vi "JSONable Tests.vi"() -> ()   [LabVIEW 2015]
uses:
  Classes/error/error.lvclass
  Classes/id/id.lvclass
  Classes/Request/Request.lvclass
  Classes/Response/Response.lvclass
  Classes/params/params.lvclass
  Classes/New folder/result.lvclass
  <vilib>/National Instruments/JSON Support for LabVIEW/JSON Data Classes/JSON String/New JSON String.vi
  <vilib>/National Instruments/JSON Support for LabVIEW/JSON Data Classes/JSON Numeric/New JSON Numeric.vi
  <vilib>/National Instruments/JSON Support for LabVIEW/JSON Data Classes/JSON Array/New JSON Array (Numeric).vi
  <vilib>/National Instruments/JSON Support for LabVIEW/JSON Data Classes/JSON Object/New JSON Object (Empty).vi
  <vilib>/National Instruments/JSON Support for LabVIEW/JSON Data Classes/JSON Object/Insert Key Value Pair (Single Boolean).vi
  <vilib>/National Instruments/JSON Support for LabVIEW/JSON Data Classes/JSON Object/Insert Key Value Pair (Single Numeric).vi
  <vilib>/National Instruments/JSON Support for LabVIEW/JSON Data Classes/JSON Object/Insert Key Value Pair (Single String).vi
  <vilib>/National Instruments/JSON Support for LabVIEW/JSON Data Classes/JSON Object/Insert Key Value Pair (Single).vi
  <vilib>/National Instruments/JSON Support for LabVIEW/JSON Data Classes/JSON Datatype/New JSON Null.vi
  Classes/JSONable/JSONable.lvclass
  <vilib>/National Instruments/JSON Support for LabVIEW/JSON Data Classes/JSON Helper/JSON Helper.lvclass
  <vilib>/National Instruments/JSON Support for LabVIEW/JSON Data Classes/JSON String/JSON String.lvclass
  <vilib>/National Instruments/JSON Support for LabVIEW/JSON Data Classes/JSON Array/JSON Array.lvclass
  <vilib>/National Instruments/JSON Support for LabVIEW/JSON Data Classes/JSON Numeric/JSON Numeric.lvclass
  <vilib>/National Instruments/JSON Support for LabVIEW/JSON Data Classes/JSON Object/JSON Object.lvclass
  <vilib>/National Instruments/JSON Support for LabVIEW/JSON Data Classes/JSON Datatype/JSON Null.lvclass
panel:
  out "result(String)":bool
  out "params(String)":bool
  out "result(named and nested)":bool
  out "result(DBL Array)":bool
  out "no result":bool
  out "response (error)":bool
  out "response (result)":bool
  out "notification":bool
  out "request (named params)":bool
  out "request (array params)":bool
  out "params(named and nested)":bool
  out "params(DBL Array)":bool
  out "no params":bool
  out "id(none)":bool
  out "id(NULL)":bool
  out "id(String)":bool
  out "id(Double)":bool
  out "error":bool
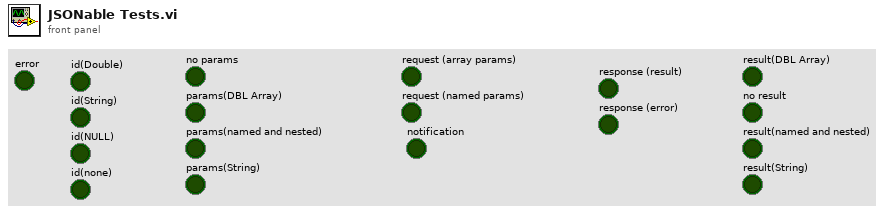
[diagram p1: front panel]
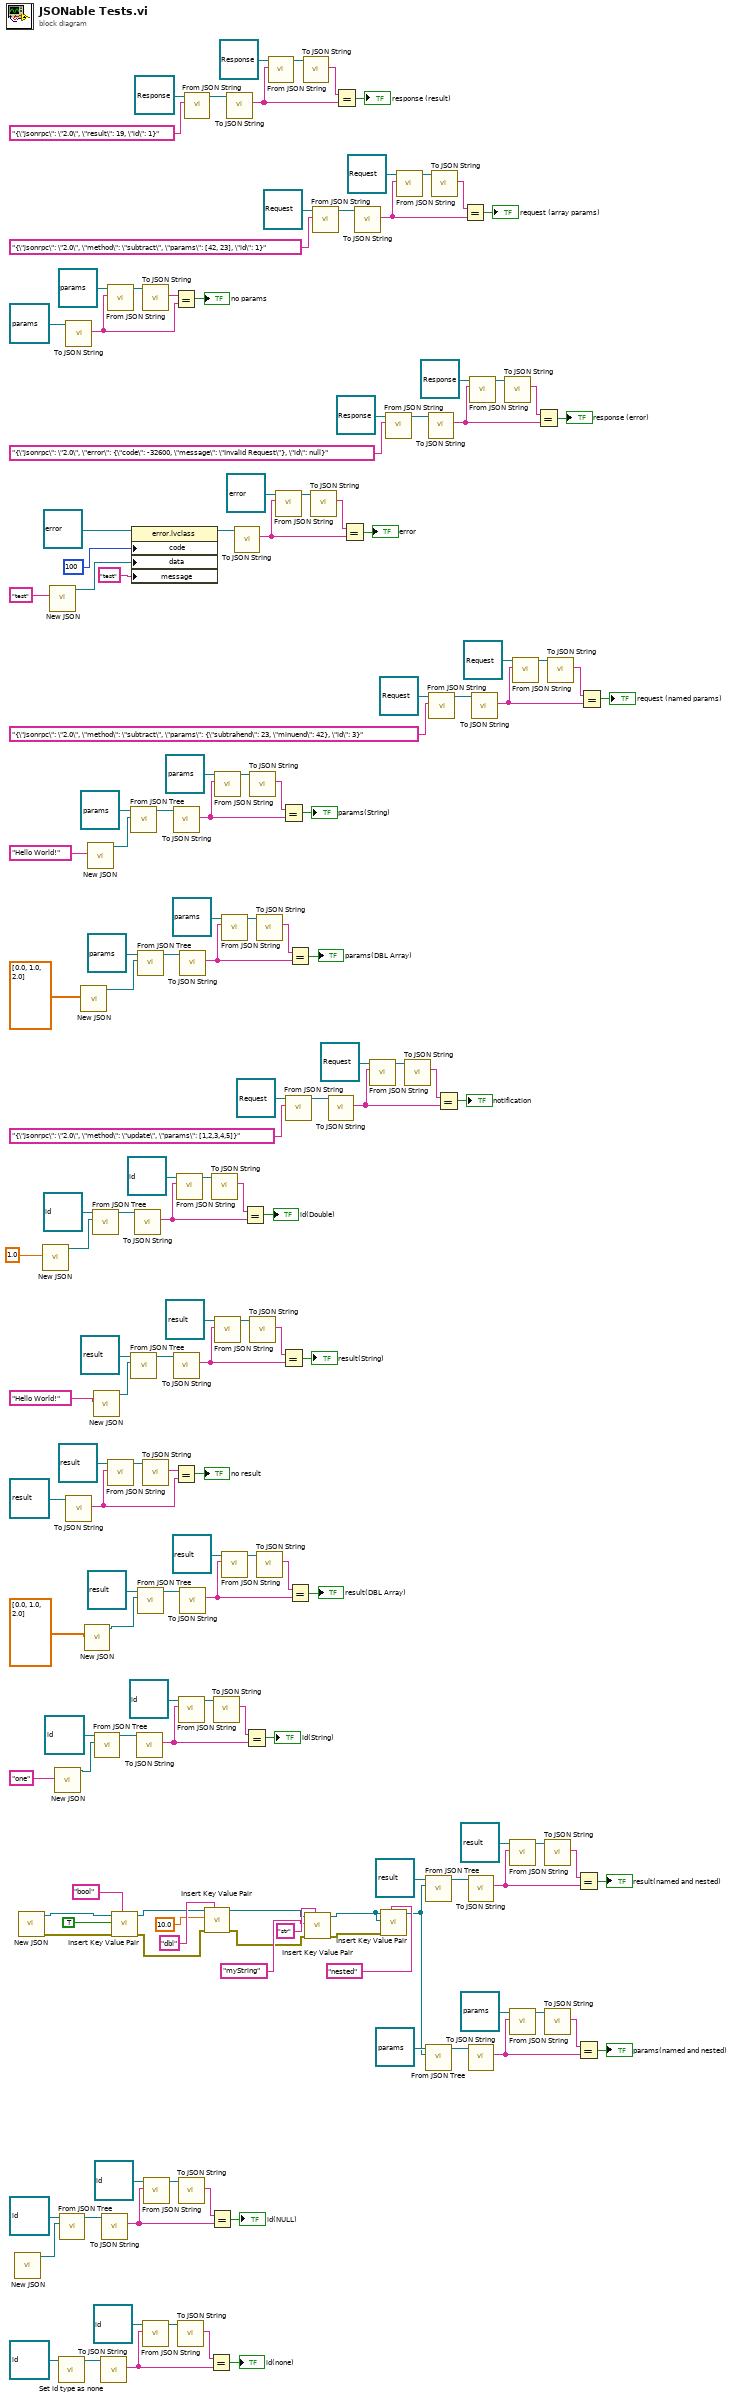
[diagram p0: block diagram]
diagram:
  n1 = call-poly <vilib>:"New JSON.vi"() -> ("JSON Null out"=w1:refnum<class "JSON Null.lvclass">)  [unwired: 10 in, 1 out]
  n2 = call-poly <vilib>:"New JSON.vi"() -> ("error out"=w14:errorcluster, "JSON Object out"=w15:refnum<class "JSON Object.lvclass">)  [unwired: 10 in]
  n3 = call-poly <vilib>:"New JSON.vi"("value"=1.0 ("Numeric")) -> ("JSON String out"=w132:refnum<class "JSON Numeric.lvclass">)  [unwired: 9 in, 1 out]
  n4 = call-poly <vilib>:"New JSON.vi"("value"="test" ("String")) -> ("JSON String out"=w145:refnum<class "JSON String.lvclass">)  [unwired: 9 in, 1 out]
  n5 = call-poly <vilib>:"New JSON.vi"("value"="one" ("String")) -> ("JSON String out"=w18:refnum<class "JSON String.lvclass">)  [unwired: 9 in, 1 out]
  n6 = call-dynamic "Set id type as none.vi"("id in"=refnum<class "id.lvclass"> refnum ("id.lvclass")) -> ("id out"=w156:refnum<class "id.lvclass">)  [unwired: 9 in, 1 out]
  n7 = call-dynamic "From JSON Tree.vi"("JSON in"=w1, "id in"=refnum<class "id.lvclass"> refnum ("id.lvclass")) -> ("id out"=w118:refnum<class "id.lvclass">)  [unwired: 8 in, 1 out]
  n8 = call "To JSON String.vi"("JSONable in"=refnum<class "params.lvclass"> refnum ("params.lvclass")) -> ("JSON String"=w154:string)  [unwired: 8 in, 2 out]
  n9 = call "To JSON String.vi"("JSONable in"=refnum<class "result.lvclass"> refnum ("result.lvclass")) -> ("JSON String"=w58:string)  [unwired: 8 in, 2 out]
  n10 = call-poly <vilib>:"New JSON.vi"("Numeric Array"=dbl[] [0.0, 1.0, 2.0] ("1D Numeric")) -> ("JSON Array out"=w110:refnum<class "JSON Array.lvclass">)  [unwired: 9 in, 1 out]
  n11 = call-poly <vilib>:"New JSON.vi"("Numeric Array"=dbl[] [0.0, 1.0, 2.0] ("1D Numeric")) -> ("JSON Array out"=w20:refnum<class "JSON Array.lvclass">)  [unwired: 9 in, 1 out]
  n12 = call-poly <vilib>:"New JSON.vi"("value"="Hello World!" ("String")) -> ("JSON String out"=w41:refnum<class "JSON String.lvclass">)  [unwired: 9 in, 1 out]
  n13 = call-dynamic "From JSON Tree.vi"("JSON in"=w132, "id in"=refnum<class "id.lvclass"> refnum ("id.lvclass")) -> ("id out"=w131:refnum<class "id.lvclass">)  [unwired: 8 in, 1 out]
  n14 = call-poly <vilib>:"New JSON.vi"("value"="Hello World!" ("String")) -> ("JSON String out"=w22:refnum<class "JSON String.lvclass">)  [unwired: 9 in, 1 out]
  n15 = call-dynamic "From JSON Tree.vi"("JSON in"=w18, "id in"=refnum<class "id.lvclass"> refnum ("id.lvclass")) -> ("id out"=w130:refnum<class "id.lvclass">)  [unwired: 8 in, 1 out]
  n16 = call "To JSON String.vi"("JSONable in"=w156) -> ("JSON String"=w159:string)  [unwired: 8 in, 2 out]
  n17 = call "To JSON String.vi"("JSONable in"=w118) -> ("JSON String"=w122:string)  [unwired: 8 in, 2 out]
  n18 = call "From JSON String.vi"("JSON String"=w154, "JSONable in"=refnum<class "params.lvclass"> refnum ("params.lvclass")) -> ("JSONable out"=w152:refnum<class "params.lvclass">)  [unwired: 8 in, 1 out]
  n19 = call "From JSON String.vi"("JSON String"=w58, "JSONable in"=refnum<class "result.lvclass"> refnum ("result.lvclass")) -> ("JSONable out"=w60:refnum<class "result.lvclass">)  [unwired: 8 in, 1 out]
  n20 = call-poly <vilib>:"Insert Key Value Pair.vi"("key"="bool" ("Name"), "error in (no error)"=w14, "value"=TRUE ("Boolean"), "JSON Object in"=w15) -> ("error out"=w10:errorcluster, "JSON Object out"=w11:refnum<class "JSON Object.lvclass">)  [unwired: 5 in, 1 out]
  n21 = call-dynamic "From JSON Tree.vi"("JSON in"=w41, "params in"=refnum<class "params.lvclass"> refnum ("params.lvclass")) -> ("params out"=w42:refnum<class "params.lvclass">)  [unwired: 8 in, 1 out]
  n22 = call-dynamic "From JSON Tree.vi"("JSON in"=w22, "result in"=refnum<class "result.lvclass"> refnum ("result.lvclass")) -> ("result out"=w27:refnum<class "result.lvclass">)  [unwired: 8 in, 1 out]
  n23 = property class="error.lvclass"(reference=refnum<class "error.lvclass"> refnum ("error.lvclass"), "code"=100, "data"=w145, "message"="test") -> (reference out=w148:refnum<class "error.lvclass">)  [unwired: 1 in, 1 out]
  n24 = call "To JSON String.vi"("JSONable in"=w131) -> ("JSON String"=w137:string)  [unwired: 8 in, 2 out]
  n25 = call "To JSON String.vi"("JSONable in"=w130) -> ("JSON String"=w125:string)  [unwired: 8 in, 2 out]
  n26 = call-dynamic "From JSON Tree.vi"("JSON in"=w110, "params in"=refnum<class "params.lvclass"> refnum ("params.lvclass")) -> ("params out"=w109:refnum<class "params.lvclass">)  [unwired: 8 in, 1 out]
  n27 = call-dynamic "From JSON Tree.vi"("JSON in"=w20, "result in"=refnum<class "result.lvclass"> refnum ("result.lvclass")) -> ("result out"=w56:refnum<class "result.lvclass">)  [unwired: 8 in, 1 out]
  n28 = call "To JSON String.vi"("JSONable in"=w152) -> ("JSON String"=w153:string)  [unwired: 8 in, 2 out]
  n29 = call "To JSON String.vi"("JSONable in"=w60) -> ("JSON String"=w59:string)  [unwired: 8 in, 2 out]
  n30 = call "From JSON String.vi"("JSON String"=w159, "JSONable in"=refnum<class "id.lvclass"> refnum ("id.lvclass")) -> ("JSONable out"=w161:refnum<class "id.lvclass">)  [unwired: 8 in, 1 out]
  n31 = call "From JSON String.vi"("JSON String"=w122, "JSONable in"=refnum<class "id.lvclass"> refnum ("id.lvclass")) -> ("JSONable out"=w120:refnum<class "id.lvclass">)  [unwired: 8 in, 1 out]
  n32 = Equal?(x=w153, y=w154) -> (x = y?=→"no params":bool)
  n33 = call "To JSON String.vi"("JSONable in"=w42) -> ("JSON String"=w38:string)  [unwired: 8 in, 2 out]
  n34 = call "To JSON String.vi"("JSONable in"=w27) -> ("JSON String"=w30:string)  [unwired: 8 in, 2 out]
  n35 = Equal?(x=w59, y=w58) -> (x = y?=→"no result":bool)
  n36 = call "From JSON String.vi"("JSON String"=w137, "JSONable in"=refnum<class "id.lvclass"> refnum ("id.lvclass")) -> ("JSONable out"=w135:refnum<class "id.lvclass">)  [unwired: 8 in, 1 out]
  n37 = call "To JSON String.vi"("JSONable in"=w161) -> ("JSON String"=w160:string)  [unwired: 8 in, 2 out]
  n38 = call "From JSON String.vi"("JSON String"=w125, "JSONable in"=refnum<class "id.lvclass"> refnum ("id.lvclass")) -> ("JSONable out"=w127:refnum<class "id.lvclass">)  [unwired: 8 in, 1 out]
  n39 = call "To JSON String.vi"("JSONable in"=w120) -> ("JSON String"=w121:string)  [unwired: 8 in, 2 out]
  n40 = call "To JSON String.vi"("JSONable in"=w109) -> ("JSON String"=w113:string)  [unwired: 8 in, 2 out]
  n41 = call "To JSON String.vi"("JSONable in"=w56) -> ("JSON String"=w53:string)  [unwired: 8 in, 2 out]
  n42 = call "From JSON String.vi"("JSON String"="{\"jsonrpc\": \"2.0\", \"result\": 19, \"id\": 1}", "JSONable in"=refnum<class "Response.lvclass"> refnum ("Response.lvclass")) -> ("JSONable out"=w77:refnum<class "Response.lvclass">)  [unwired: 8 in, 1 out]
  n43 = call-poly <vilib>:"Insert Key Value Pair.vi"("key"="dbl" ("Name"), "error in (no error)"=w10, "value"=10.0 ("Numeric"), "JSON Object in"=w11) -> ("error out"=w7:errorcluster, "JSON Object out"=w5:refnum<class "JSON Object.lvclass">)  [unwired: 5 in, 1 out]
  n44 = Equal?(x=w160, y=w159) -> (x = y?=→"id(none)":bool)
  n45 = Equal?(x=w121, y=w122) -> (x = y?=→"id(NULL)":bool)
  n46 = call "To JSON String.vi"("JSONable in"=w135) -> ("JSON String"=w136:string)  [unwired: 8 in, 2 out]
  n47 = call "To JSON String.vi"("JSONable in"=w127) -> ("JSON String"=w126:string)  [unwired: 8 in, 2 out]
  n48 = call "From JSON String.vi"("JSON String"=w38, "JSONable in"=refnum<class "params.lvclass"> refnum ("params.lvclass")) -> ("JSONable out"=w36:refnum<class "params.lvclass">)  [unwired: 8 in, 1 out]
  n49 = call "From JSON String.vi"("JSON String"=w30, "JSONable in"=refnum<class "result.lvclass"> refnum ("result.lvclass")) -> ("JSONable out"=w32:refnum<class "result.lvclass">)  [unwired: 8 in, 1 out]
  n50 = call "From JSON String.vi"("JSON String"=w113, "JSONable in"=refnum<class "params.lvclass"> refnum ("params.lvclass")) -> ("JSONable out"=w115:refnum<class "params.lvclass">)  [unwired: 8 in, 1 out]
  n51 = call "From JSON String.vi"("JSON String"=w53, "JSONable in"=refnum<class "result.lvclass"> refnum ("result.lvclass")) -> ("JSONable out"=w51:refnum<class "result.lvclass">)  [unwired: 8 in, 1 out]
  n52 = call "To JSON String.vi"("JSONable in"=w77) -> ("JSON String"=w72:string)  [unwired: 8 in, 2 out]
  n53 = call "To JSON String.vi"("JSONable in"=w148) -> ("JSON String"=w140:string)  [unwired: 8 in, 2 out]
  n54 = Equal?(x=w136, y=w137) -> (x = y?=→"id(Double)":bool)
  n55 = Equal?(x=w126, y=w125) -> (x = y?=→"id(String)":bool)
  n56 = call "To JSON String.vi"("JSONable in"=w36) -> ("JSON String"=w37:string)  [unwired: 8 in, 2 out]
  n57 = call "To JSON String.vi"("JSONable in"=w32) -> ("JSON String"=w31:string)  [unwired: 8 in, 2 out]
  n58 = call "To JSON String.vi"("JSONable in"=w115) -> ("JSON String"=w114:string)  [unwired: 8 in, 2 out]
  n59 = call "To JSON String.vi"("JSONable in"=w51) -> ("JSON String"=w52:string)  [unwired: 8 in, 2 out]
  n60 = call "From JSON String.vi"("JSON String"=w72, "JSONable in"=refnum<class "Response.lvclass"> refnum ("Response.lvclass")) -> ("JSONable out"=w74:refnum<class "Response.lvclass">)  [unwired: 8 in, 1 out]
  n61 = call "From JSON String.vi"("JSON String"=w140, "JSONable in"=refnum<class "error.lvclass"> refnum ("error.lvclass")) -> ("JSONable out"=w142:refnum<class "error.lvclass">)  [unwired: 8 in, 1 out]
  n62 = Equal?(x=w37, y=w38) -> (x = y?=→"params(String)":bool)
  n63 = Equal?(x=w31, y=w30) -> (x = y?=→"result(String)":bool)
  n64 = call "From JSON String.vi"("JSON String"="{\"jsonrpc\": \"2.0\", \"method\": \"update\", \"params\": [1,2,3,4,5]}", "JSONable in"=refnum<class "Request.lvclass"> refnum ("Request.lvclass")) -> ("JSONable out"=w80:refnum<class "Request.lvclass">)  [unwired: 8 in, 1 out]
  n65 = Equal?(x=w114, y=w113) -> (x = y?=→"params(DBL Array)":bool)
  n66 = Equal?(x=w52, y=w53) -> (x = y?=→"result(DBL Array)":bool)
  n67 = call "To JSON String.vi"("JSONable in"=w74) -> ("JSON String"=w73:string)  [unwired: 8 in, 2 out]
  n68 = call-poly <vilib>:"Insert Key Value Pair.vi"("key"="str" ("Name"), "error in (no error)"=w7, "value"="myString" ("String"), "JSON Object in"=w5) -> ("error out"=w6:errorcluster, "JSON Object out"=w4:refnum<class "JSON Object.lvclass">)  [unwired: 5 in, 1 out]
  n69 = call "To JSON String.vi"("JSONable in"=w142) -> ("JSON String"=w141:string)  [unwired: 8 in, 2 out]
  n70 = call "From JSON String.vi"("JSON String"="{\"jsonrpc\": \"2.0\", \"method\": \"subtract\", \"params\": [42, 23], \"id\": 1}", "JSONable in"=refnum<class "Request.lvclass"> refnum ("Request.lvclass")) -> ("JSONable out"=w95:refnum<class "Request.lvclass">)  [unwired: 8 in, 1 out]
  n71 = call "To JSON String.vi"("JSONable in"=w80) -> ("JSON String"=w85:string)  [unwired: 8 in, 2 out]
  n72 = Equal?(x=w73, y=w72) -> (x = y?=→"response (result)":bool)
  n73 = Equal?(x=w141, y=w140) -> (x = y?=→"error":bool)
  n74 = call "To JSON String.vi"("JSONable in"=w95) -> ("JSON String"=w100:string)  [unwired: 8 in, 2 out]
  n75 = call "From JSON String.vi"("JSON String"=w85, "JSONable in"=refnum<class "Request.lvclass"> refnum ("Request.lvclass")) -> ("JSONable out"=w83:refnum<class "Request.lvclass">)  [unwired: 8 in, 1 out]
  n76 = call-poly <vilib>:"Insert Key Value Pair.vi"("key"="nested" ("Name"), "error in (no error)"=w6, "value"=w4, "JSON Object in"=w4) -> ("JSON Object out"=w2:refnum<class "JSON Object.lvclass">)  [unwired: 5 in, 2 out]
  n77 = call "From JSON String.vi"("JSON String"="{\"jsonrpc\": \"2.0\", \"error\": {\"code\": -32600, \"message\": \"Invalid Request\"}, \"id\": null}", "JSONable in"=refnum<class "Response.lvclass"> refnum ("Response.lvclass")) -> ("JSONable out"=w64:refnum<class "Response.lvclass">)  [unwired: 8 in, 1 out]
  n78 = call "From JSON String.vi"("JSON String"=w100, "JSONable in"=refnum<class "Request.lvclass"> refnum ("Request.lvclass")) -> ("JSONable out"=w98:refnum<class "Request.lvclass">)  [unwired: 8 in, 1 out]
  n79 = call "To JSON String.vi"("JSONable in"=w83) -> ("JSON String"=w84:string)  [unwired: 8 in, 2 out]
  n80 = call-dynamic "From JSON Tree.vi"("JSON in"=w2, "result in"=refnum<class "result.lvclass"> refnum ("result.lvclass")) -> ("result out"=w43:refnum<class "result.lvclass">)  [unwired: 8 in, 1 out]
  n81 = call-dynamic "From JSON Tree.vi"("JSON in"=w2, "params in"=refnum<class "params.lvclass"> refnum ("params.lvclass")) -> ("params out"=w108:refnum<class "params.lvclass">)  [unwired: 8 in, 1 out]
  n82 = call "To JSON String.vi"("JSONable in"=w64) -> ("JSON String"=w69:string)  [unwired: 8 in, 2 out]
  n83 = call "From JSON String.vi"("JSON String"="{\"jsonrpc\": \"2.0\", \"method\": \"subtract\", \"params\": {\"subtrahend\": 23, \"minuend\": 42}, \"id\": 3}", "JSONable in"=refnum<class "Request.lvclass"> refnum ("Request.lvclass")) -> ("JSONable out"=w26:refnum<class "Request.lvclass">)  [unwired: 8 in, 1 out]
  n84 = call "To JSON String.vi"("JSONable in"=w98) -> ("JSON String"=w99:string)  [unwired: 8 in, 2 out]
  n85 = Equal?(x=w84, y=w85) -> (x = y?=→"notification":bool)
  n86 = Equal?(x=w99, y=w100) -> (x = y?=→"request (array params)":bool)
  n87 = call "To JSON String.vi"("JSONable in"=w43) -> ("JSON String"=w46:string)  [unwired: 8 in, 2 out]
  n88 = call "To JSON String.vi"("JSONable in"=w108) -> ("JSON String"=w105:string)  [unwired: 8 in, 2 out]
  n89 = call "From JSON String.vi"("JSON String"=w69, "JSONable in"=refnum<class "Response.lvclass"> refnum ("Response.lvclass")) -> ("JSONable out"=w67:refnum<class "Response.lvclass">)  [unwired: 8 in, 1 out]
  n90 = call "To JSON String.vi"("JSONable in"=w26) -> ("JSON String"=w88:string)  [unwired: 8 in, 2 out]
  n91 = call "To JSON String.vi"("JSONable in"=w67) -> ("JSON String"=w68:string)  [unwired: 8 in, 2 out]
  n92 = call "From JSON String.vi"("JSON String"=w46, "JSONable in"=refnum<class "result.lvclass"> refnum ("result.lvclass")) -> ("JSONable out"=w48:refnum<class "result.lvclass">)  [unwired: 8 in, 1 out]
  n93 = call "From JSON String.vi"("JSON String"=w105, "JSONable in"=refnum<class "params.lvclass"> refnum ("params.lvclass")) -> ("JSONable out"=w103:refnum<class "params.lvclass">)  [unwired: 8 in, 1 out]
  n94 = call "From JSON String.vi"("JSON String"=w88, "JSONable in"=refnum<class "Request.lvclass"> refnum ("Request.lvclass")) -> ("JSONable out"=w90:refnum<class "Request.lvclass">)  [unwired: 8 in, 1 out]
  n95 = Equal?(x=w68, y=w69) -> (x = y?=→"response (error)":bool)
  n96 = call "To JSON String.vi"("JSONable in"=w48) -> ("JSON String"=w47:string)  [unwired: 8 in, 2 out]
  n97 = call "To JSON String.vi"("JSONable in"=w103) -> ("JSON String"=w104:string)  [unwired: 8 in, 2 out]
  n98 = call "To JSON String.vi"("JSONable in"=w90) -> ("JSON String"=w89:string)  [unwired: 8 in, 2 out]
  n99 = Equal?(x=w47, y=w46) -> (x = y?=→"result(named and nested)":bool)
  n100 = Equal?(x=w104, y=w105) -> (x = y?=→"params(named and nested)":bool)
  n101 = Equal?(x=w89, y=w88) -> (x = y?=→"request (named params)":bool)
